vi "cl_serv_serv.vi"() -> ()   [LabVIEW 2015]
panel:
  out "String":string
  in  "close connection 4":bool
  in  "Control 4":bool
  in  "Slide 4":dbl(slide) scale=0.0..10.0
  out "number 4":dbl(slide) scale=0.0..10.0
  out "name:port 4":string
  out "ip:port23":string
  in  "close server 4":bool
  in  "Server Closed 4":string="The server VI closed the connection."
  in  "close connection 3":bool
  in  "Control 3":bool
  in  "Slide 3":dbl(slide) scale=0.0..10.0
  out "number 3":dbl(slide) scale=0.0..10.0
  out "name:port 3":string
  out "ip:port2 2":string
  in  "close server 3":bool
  in  "Server Closed 3":string="The server VI closed the connection."
  in  "close connection 2":bool
  in  "Control 2":bool
  in  "Slide 2":dbl(slide) scale=0.0..10.0
  out "number 2":dbl(slide) scale=0.0..10.0
  out "name:port 2":string
  out "ip:port2":string
  in  "close server 2":bool
  in  "Server Closed 2":string="The server VI closed the connection."
  in  "close server 1":bool
  out "ip:port 1":string
  out "name:port 1":string
  out "number 1":dbl(slide) scale=0.0..10.0
  in  "Slide 1":dbl(slide) scale=0.0..10.0
  in  "Control 1":bool
  in  "Server Closed 1":string="The server VI closed the connection."
  in  "close connection":bool
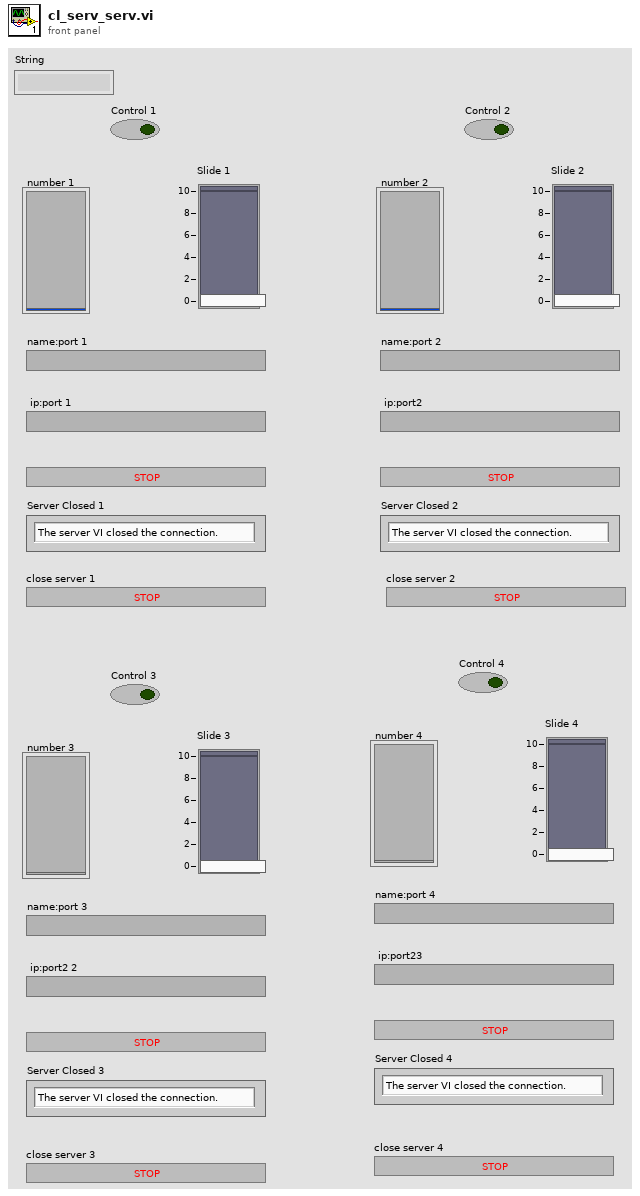
[diagram p1: front panel]
types:
  T1 = enum8{"Enabled", "Disabled", "Disabled and Grayed Out"}
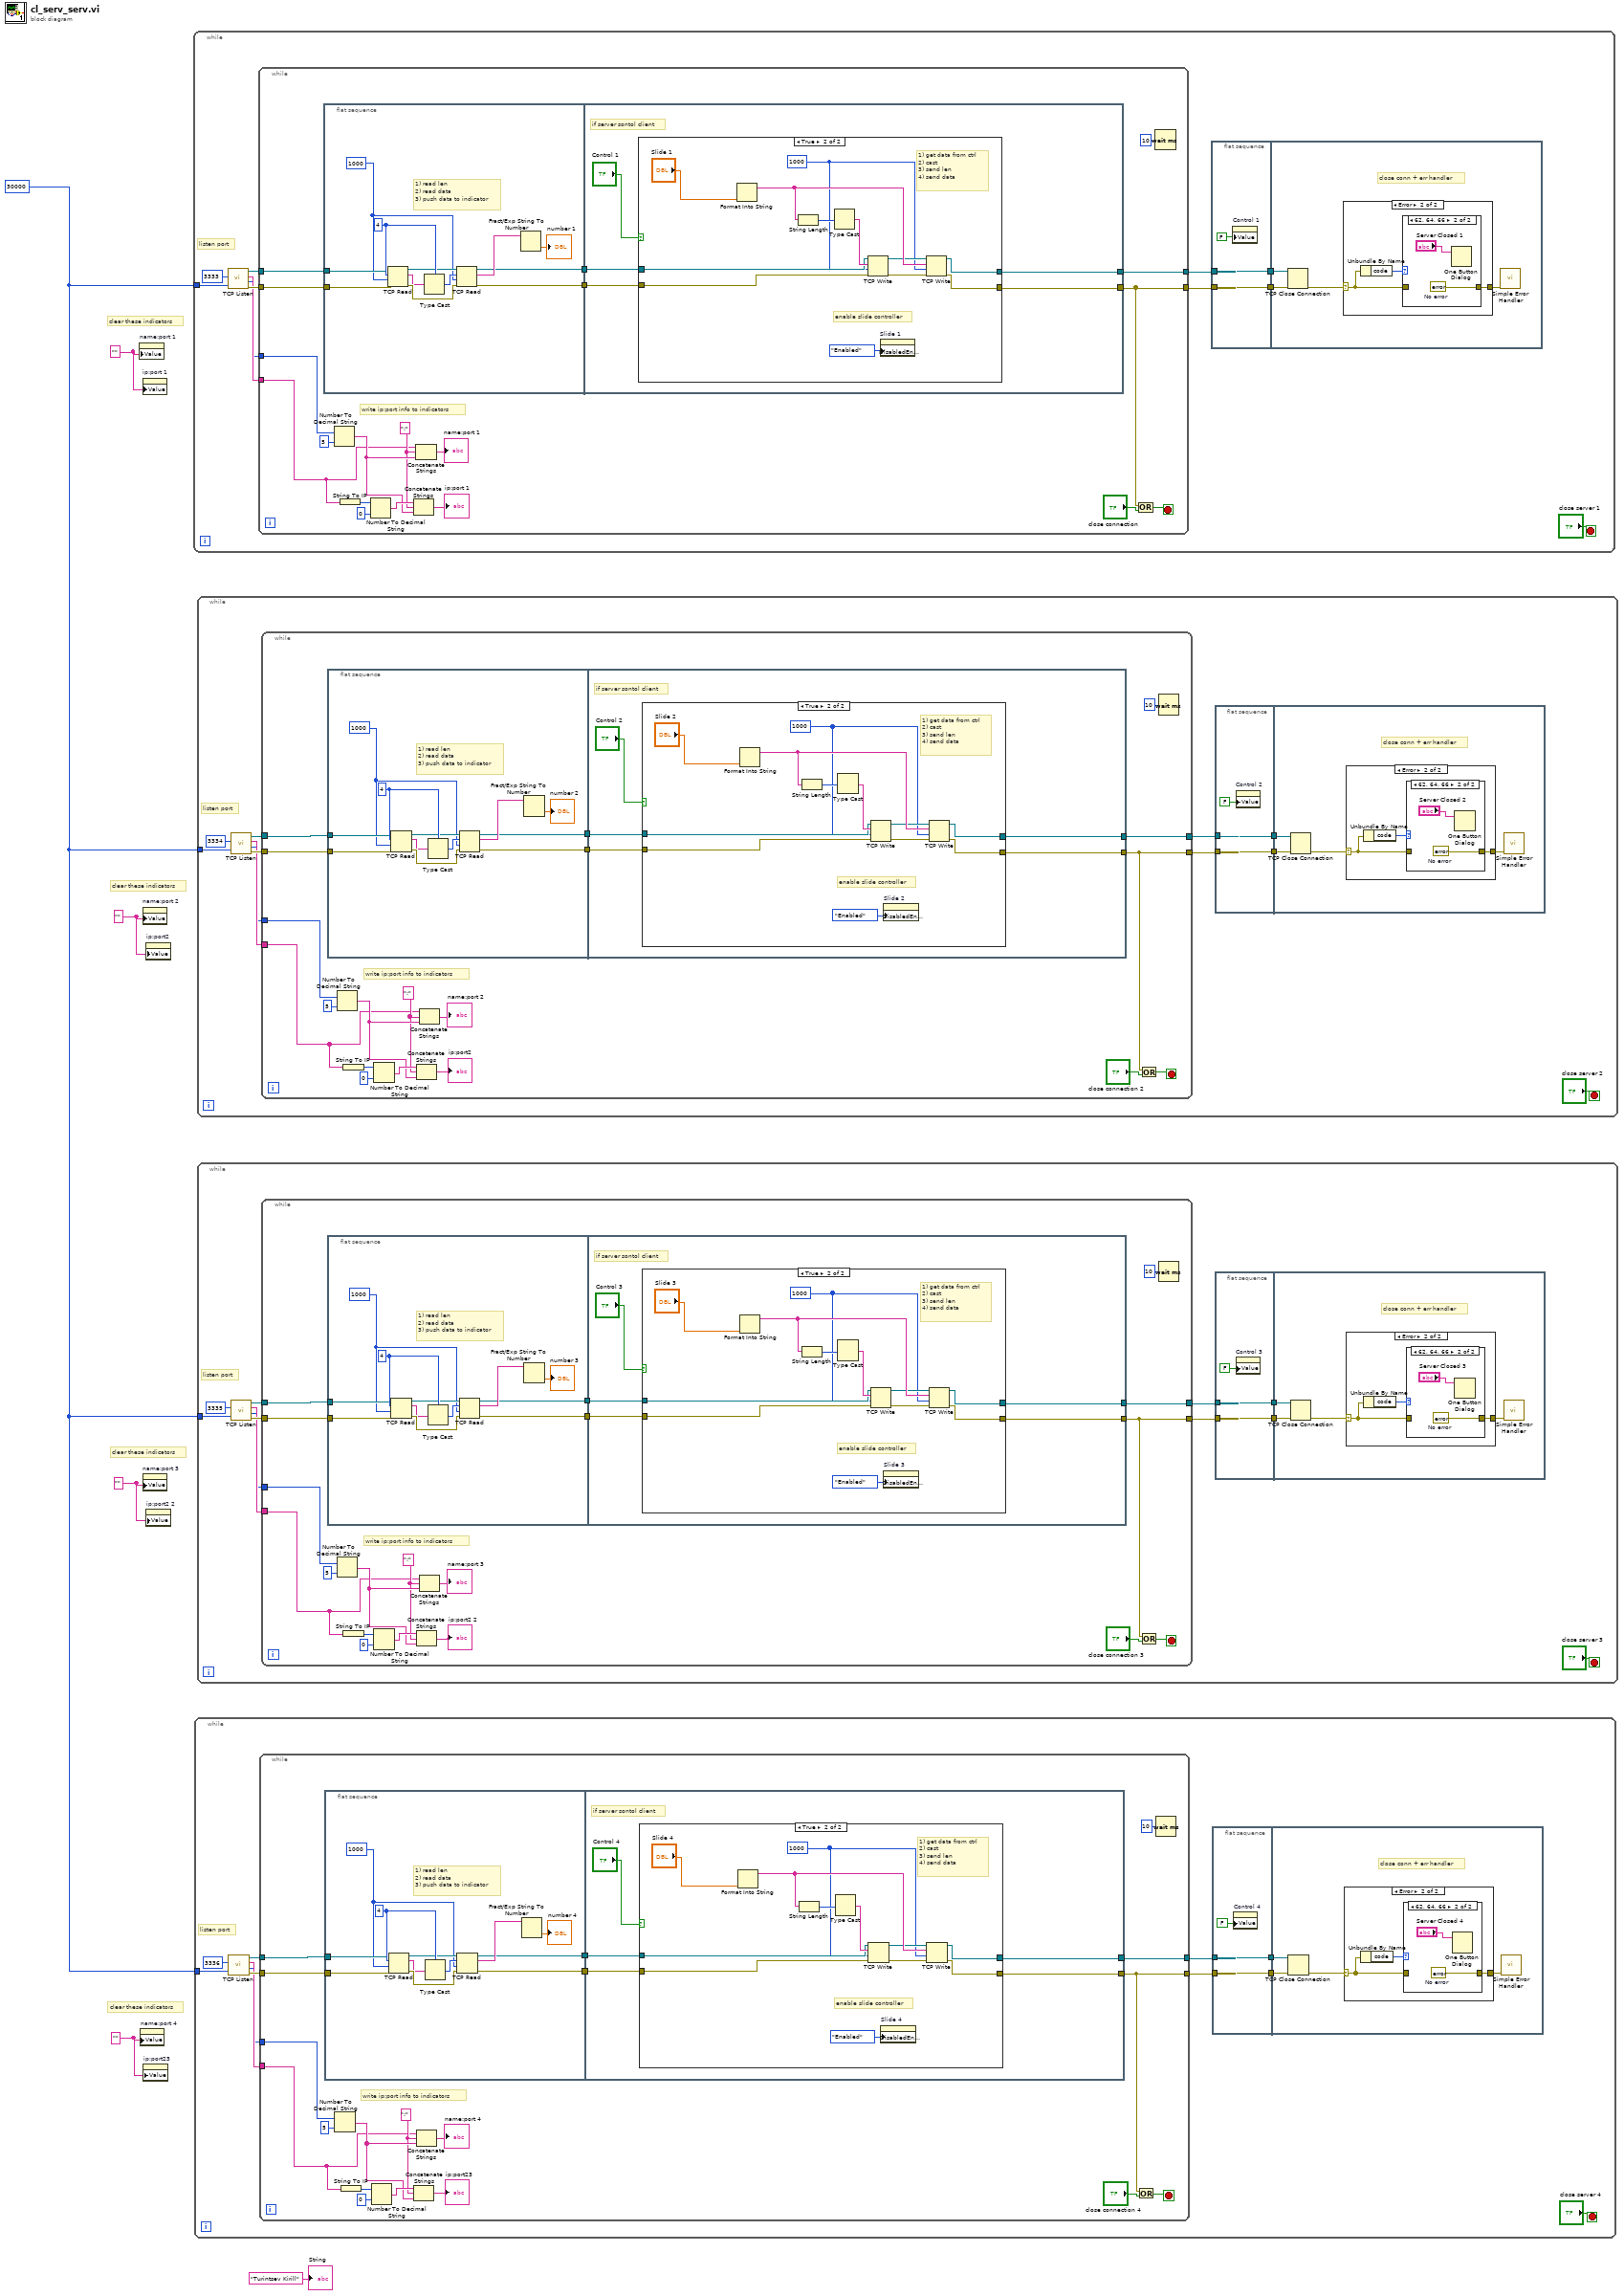
[diagram p0: block diagram]
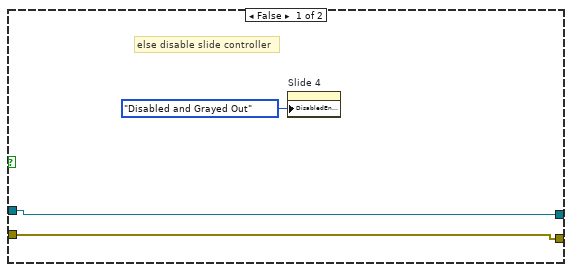
[diagram p4: hidden frame]
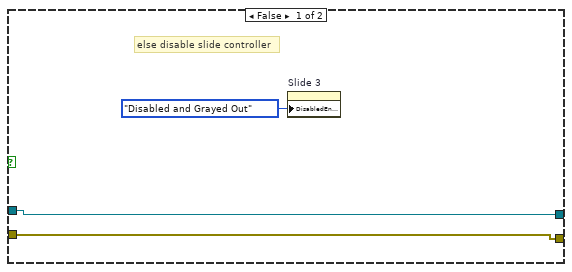
[diagram p7: hidden frame]
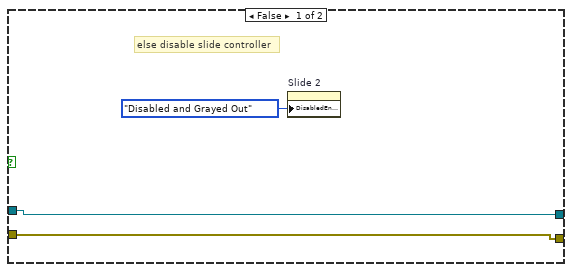
[diagram p10: hidden frame]
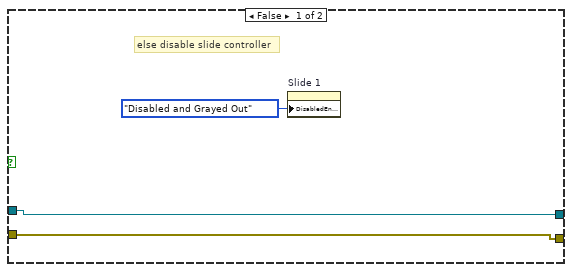
[diagram p13: hidden frame]
diagram:
  w3 = "" ("name:port 1")
  w4 = "" ("name:port 1")
  w5 = "" ("name:port 1")
  w2 = 30000 ("timeout ms (wait forever: -1)")
  w6 = "" ("name:port 1")
  # "clear these indicators"
  # "clear these indicators"
  # "clear these indicators"
  # "clear these indicators"
  n1 = property on="name:port 1" class="Str"("Value"=w6) -> ()  [unwired: 2 in, 2 out]
  n2 = property on="name:port 4" class="Str"("Value"=w3) -> ()  [unwired: 2 in, 2 out]
  n3 = property on="ip:port 1" class="Str"("Value"=w6) -> ()  [unwired: 2 in, 2 out]
  n4 = property on="name:port 2" class="Str"("Value"=w5) -> ()  [unwired: 2 in, 2 out]
  n5 = property on="name:port 3" class="Str"("Value"=w4) -> ()  [unwired: 2 in, 2 out]
  n6 = property on="ip:port23" class="Str"("Value"=w3) -> ()  [unwired: 2 in, 2 out]
  n7 = property on="ip:port2" class="Str"("Value"=w5) -> ()  [unwired: 2 in, 2 out]
  n8 = property on="ip:port2 2" class="Str"("Value"=w4) -> ()  [unwired: 2 in, 2 out]
  n9 = while {
    tunnel: w2 -> [w10]
    stop <- "close server 1" stop-if-true
    # "listen port"
    n10 = call <vilib>:"TCP Listen.vi"("timeout ms (wait forever: -1)"=w10, "port"=u16 3333) -> ("error out"=w14:errorcluster, "remote port"=w11:u16, "remote address"=w12:string, "connection ID"=w16:refnum<k5>)  [unwired: 5 in, 1 out]
    n11 = while {
      tunnel: w16 -> [w50]
      tunnel: [w46] -> w15
      tunnel: w14 -> [w49]
      tunnel: [w32] -> w13
      tunnel: w12 -> [w37]
      tunnel: w11 -> [w36]
      stop <- w34 stop-if-true
      w38 = ":" ("string")
      # "write ip:port info to indicators"
      n12 = flat-sequence {
        tunnel: w50 -> [w55]
        tunnel: w49 -> [w54]
        tunnel: [w53] -> w48
        tunnel: [w52] -> w47
        tunnel: w48 -> [w66]
        tunnel: w47 -> [w65]
        tunnel: [w64] -> w46
        tunnel: [w63] -> w32
        frame #0 {
          w51 = 1000 ("timeout ms (25000)")
          w59 = 4 ("bytes to read")
          # "1) read len\n2) read data\n3) push data to indicator"
          n13 = TCP Read(connection ID=w55, bytes to read=w59, error in (no error)=w54, 9:w51) -> (connection ID out=w56:refnum<k5>, data out=w57:string, error out=w60:errorcluster)  [unwired: 1 in]
          n14 = Type Cast(type=w59, x=w57) -> (*(type *) &x=w58:i32)
          n15 = TCP Read(connection ID=w56, bytes to read=w58, error in (no error)=w60, 9:w51) -> (connection ID out=w53:refnum<k5>, data out=w61:string, error out=w52:errorcluster)  [unwired: 1 in]
          n16 = Fract/Exp String To Number(string=w61) -> (number=→"number 1":dbl)  [unwired: 3 in, 1 out]
        }
        frame #1 {
          # "if server sontol client"
          n17 = case shown="True" "Control 1" {
            tunnel: w66 -> [w70 w76]
            tunnel: w65 -> [w69 w75]
            tunnel: [w70 w74] -> w64
            tunnel: [w69 w73] -> w63
            frame False {
              # "else disable slide controller"
              n18 = property on="Slide 1" class="Slide (strict)"("DisabledEnum"=T1."Disabled and Grayed Out" ("Disabled")) -> ()  [unwired: 2 in, 2 out]
            }
            frame True {
              w71 = 1000 ("timeout ms (25000)")
              # "1) get data from ctrl\n2) cast\n3) send len\n4) send data"
              # "enable slide controller"
              n19 = Format Into String("Slide 1") -> (resulting string=w82:string)  [unwired: 3 in, 1 out]
              n20 = String Length(string=w82) -> (length=w79:i32)
              n21 = Type Cast(x=w79) -> (*(type *) &x=w80:string)  [unwired: 1 out]
              n22 = TCP Write(connection ID=w76, data in=w80, error in (no error)=w75, 9:w71) -> (connection ID out=w77:refnum<k5>, error out=w78:errorcluster)  [unwired: 1 out]
              n23 = property on="Slide 1" class="Slide (strict)"("DisabledEnum"=T1."Enabled" ("Disabled")) -> ()  [unwired: 2 in, 2 out]
              n24 = TCP Write(connection ID=w77, data in=w82, error in (no error)=w78, 9:w71) -> (connection ID out=w74:refnum<k5>, error out=w73:errorcluster)  [unwired: 1 out]
            }
          }
        }
      }
      n25 = Number To Decimal String(number=w36, width (-)=i16 5) -> (decimal integer string=w40:string)
      n26 = String To IP(1:w37) -> (0:w43:u32)
      n27 = Number To Decimal String(number=w43, width (-)=i16 0) -> (decimal integer string=w41:string)
      n28 = Concatenate Strings(w41, w38, w40) -> (→"ip:port 1":string)
      n29 = Concatenate Strings(w37, w38, w40) -> (→"name:port 1":string)
      n30 = Or(x=w32, y="close connection") -> (x .or. y?=w34:bool)
      n31 = Wait (ms)(milliseconds to wait=u32 10) -> ()  [unwired: 1 out]
    }
    n32 = flat-sequence {
      tunnel: w13 -> [w19]
      tunnel: w15 -> [w20]
      tunnel: [w20] -> w8
      tunnel: [w19] -> w7
      tunnel: w8 -> [w24]
      tunnel: w7 -> [w22]
      frame #0 {
        n33 = property on="Control 1" class="Bool (strict)"("Value"=FALSE ("Control 1")) -> ()  [unwired: 2 in, 2 out]
      }
      frame #1 {
        # "close conn + err handler"
        n34 = TCP Close Connection(connection ID=w24, error in (no error)=w22) -> (error out=w21:errorcluster)  [unwired: 1 in, 1 out]
        n35 = case shown="Error" w21 {
          selector: w21 -> [w25 w27]
          tunnel: [w25 w26] -> w23
          frame No Error {
          }
          frame Error {
            n36 = Unbundle By Name(w27) -> ("code"=w28:i32)
            n37 = case shown="62, 64, 66" w28 {
              tunnel: w27 -> [w29 _]
              tunnel: [w29 w31] -> w26
              frame Default {
              }
              frame 62, 64, 66 {
                w31 = errorcluster {"status"=FALSE, "code"=0, "source"=""}  # No error
                n38 = One Button Dialog(message="Server Closed 1") -> ()  [unwired: 1 in, 1 out]
              }
            }
          }
        }
        n39 = call <vilib>:"Simple Error Handler.vi"("error in (no error)"=w23) -> ()  [unwired: 1 in, 8 out]
      }
    }
  }
  n40 = while {
    tunnel: w2 -> [w86]
    stop <- "close server 4" stop-if-true
    # "listen port"
    n41 = call <vilib>:"TCP Listen.vi"("timeout ms (wait forever: -1)"=w86, "port"=u16 3336) -> ("error out"=w90:errorcluster, "remote port"=w87:u16, "remote address"=w88:string, "connection ID"=w92:refnum<k5>)  [unwired: 5 in, 1 out]
    n42 = while {
      tunnel: w92 -> [w126]
      tunnel: [w122] -> w91
      tunnel: w90 -> [w125]
      tunnel: [w108] -> w89
      tunnel: w88 -> [w113]
      tunnel: w87 -> [w112]
      stop <- w110 stop-if-true
      w114 = ":" ("string")
      # "write ip:port info to indicators"
      n43 = flat-sequence {
        tunnel: w126 -> [w131]
        tunnel: w125 -> [w130]
        tunnel: [w129] -> w124
        tunnel: [w128] -> w123
        tunnel: w124 -> [w142]
        tunnel: w123 -> [w141]
        tunnel: [w140] -> w122
        tunnel: [w139] -> w108
        frame #0 {
          w127 = 1000 ("timeout ms (25000)")
          w135 = 4 ("bytes to read")
          # "1) read len\n2) read data\n3) push data to indicator"
          n44 = TCP Read(connection ID=w131, bytes to read=w135, error in (no error)=w130, 9:w127) -> (connection ID out=w132:refnum<k5>, data out=w133:string, error out=w136:errorcluster)  [unwired: 1 in]
          n45 = Type Cast(type=w135, x=w133) -> (*(type *) &x=w134:i32)
          n46 = TCP Read(connection ID=w132, bytes to read=w134, error in (no error)=w136, 9:w127) -> (connection ID out=w129:refnum<k5>, data out=w137:string, error out=w128:errorcluster)  [unwired: 1 in]
          n47 = Fract/Exp String To Number(string=w137) -> (number=→"number 4":dbl)  [unwired: 3 in, 1 out]
        }
        frame #1 {
          # "if server sontol client"
          n48 = case shown="True" "Control 4" {
            tunnel: w142 -> [w146 w152]
            tunnel: w141 -> [w145 w151]
            tunnel: [w146 w150] -> w140
            tunnel: [w145 w149] -> w139
            frame False {
              # "else disable slide controller"
              n49 = property on="Slide 4" class="Slide (strict)"("DisabledEnum"=T1."Disabled and Grayed Out" ("Disabled")) -> ()  [unwired: 2 in, 2 out]
            }
            frame True {
              w147 = 1000 ("timeout ms (25000)")
              # "1) get data from ctrl\n2) cast\n3) send len\n4) send data"
              # "enable slide controller"
              n50 = Format Into String("Slide 4") -> (resulting string=w158:string)  [unwired: 3 in, 1 out]
              n51 = String Length(string=w158) -> (length=w155:i32)
              n52 = Type Cast(x=w155) -> (*(type *) &x=w156:string)  [unwired: 1 out]
              n53 = TCP Write(connection ID=w152, data in=w156, error in (no error)=w151, 9:w147) -> (connection ID out=w153:refnum<k5>, error out=w154:errorcluster)  [unwired: 1 out]
              n54 = property on="Slide 4" class="Slide (strict)"("DisabledEnum"=T1."Enabled" ("Disabled")) -> ()  [unwired: 2 in, 2 out]
              n55 = TCP Write(connection ID=w153, data in=w158, error in (no error)=w154, 9:w147) -> (connection ID out=w150:refnum<k5>, error out=w149:errorcluster)  [unwired: 1 out]
            }
          }
        }
      }
      n56 = Number To Decimal String(number=w112, width (-)=i16 5) -> (decimal integer string=w116:string)
      n57 = String To IP(1:w113) -> (0:w119:u32)
      n58 = Number To Decimal String(number=w119, width (-)=i16 0) -> (decimal integer string=w117:string)
      n59 = Concatenate Strings(w117, w114, w116) -> (→"ip:port23":string)
      n60 = Concatenate Strings(w113, w114, w116) -> (→"name:port 4":string)
      n61 = Or(x=w108, y="close connection 4") -> (x .or. y?=w110:bool)
      n62 = Wait (ms)(milliseconds to wait=u32 10) -> ()  [unwired: 1 out]
    }
    n63 = flat-sequence {
      tunnel: w89 -> [w95]
      tunnel: w91 -> [w96]
      tunnel: [w96] -> w84
      tunnel: [w95] -> w83
      tunnel: w84 -> [w100]
      tunnel: w83 -> [w98]
      frame #0 {
        n64 = property on="Control 4" class="Bool (strict)"("Value"=FALSE ("Control 1")) -> ()  [unwired: 2 in, 2 out]
      }
      frame #1 {
        # "close conn + err handler"
        n65 = TCP Close Connection(connection ID=w100, error in (no error)=w98) -> (error out=w97:errorcluster)  [unwired: 1 in, 1 out]
        n66 = case shown="Error" w97 {
          selector: w97 -> [w101 w103]
          tunnel: [w101 w102] -> w99
          frame No Error {
          }
          frame Error {
            n67 = Unbundle By Name(w103) -> ("code"=w104:i32)
            n68 = case shown="62, 64, 66" w104 {
              tunnel: w103 -> [w105 _]
              tunnel: [w105 w107] -> w102
              frame Default {
              }
              frame 62, 64, 66 {
                w107 = errorcluster {"status"=FALSE, "code"=0, "source"=""}  # No error
                n69 = One Button Dialog(message="Server Closed 4") -> ()  [unwired: 1 in, 1 out]
              }
            }
          }
        }
        n70 = call <vilib>:"Simple Error Handler.vi"("error in (no error)"=w99) -> ()  [unwired: 1 in, 8 out]
      }
    }
  }
  n71 = while {
    tunnel: w2 -> [w162]
    stop <- "close server 2" stop-if-true
    # "listen port"
    n72 = call <vilib>:"TCP Listen.vi"("timeout ms (wait forever: -1)"=w162, "port"=u16 3334) -> ("error out"=w166:errorcluster, "remote port"=w163:u16, "remote address"=w164:string, "connection ID"=w168:refnum<k5>)  [unwired: 5 in, 1 out]
    n73 = while {
      tunnel: w168 -> [w202]
      tunnel: [w198] -> w167
      tunnel: w166 -> [w201]
      tunnel: [w184] -> w165
      tunnel: w164 -> [w189]
      tunnel: w163 -> [w188]
      stop <- w186 stop-if-true
      w190 = ":" ("string")
      # "write ip:port info to indicators"
      n74 = flat-sequence {
        tunnel: w202 -> [w207]
        tunnel: w201 -> [w206]
        tunnel: [w205] -> w200
        tunnel: [w204] -> w199
        tunnel: w200 -> [w218]
        tunnel: w199 -> [w217]
        tunnel: [w216] -> w198
        tunnel: [w215] -> w184
        frame #0 {
          w203 = 1000 ("timeout ms (25000)")
          w211 = 4 ("bytes to read")
          # "1) read len\n2) read data\n3) push data to indicator"
          n75 = TCP Read(connection ID=w207, bytes to read=w211, error in (no error)=w206, 9:w203) -> (connection ID out=w208:refnum<k5>, data out=w209:string, error out=w212:errorcluster)  [unwired: 1 in]
          n76 = Type Cast(type=w211, x=w209) -> (*(type *) &x=w210:i32)
          n77 = TCP Read(connection ID=w208, bytes to read=w210, error in (no error)=w212, 9:w203) -> (connection ID out=w205:refnum<k5>, data out=w213:string, error out=w204:errorcluster)  [unwired: 1 in]
          n78 = Fract/Exp String To Number(string=w213) -> (number=→"number 2":dbl)  [unwired: 3 in, 1 out]
        }
        frame #1 {
          # "if server sontol client"
          n79 = case shown="True" "Control 2" {
            tunnel: w218 -> [w222 w228]
            tunnel: w217 -> [w221 w227]
            tunnel: [w222 w226] -> w216
            tunnel: [w221 w225] -> w215
            frame False {
              # "else disable slide controller"
              n80 = property on="Slide 2" class="Slide (strict)"("DisabledEnum"=T1."Disabled and Grayed Out" ("Disabled")) -> ()  [unwired: 2 in, 2 out]
            }
            frame True {
              w223 = 1000 ("timeout ms (25000)")
              # "1) get data from ctrl\n2) cast\n3) send len\n4) send data"
              # "enable slide controller"
              n81 = Format Into String("Slide 2") -> (resulting string=w234:string)  [unwired: 3 in, 1 out]
              n82 = String Length(string=w234) -> (length=w231:i32)
              n83 = Type Cast(x=w231) -> (*(type *) &x=w232:string)  [unwired: 1 out]
              n84 = TCP Write(connection ID=w228, data in=w232, error in (no error)=w227, 9:w223) -> (connection ID out=w229:refnum<k5>, error out=w230:errorcluster)  [unwired: 1 out]
              n85 = property on="Slide 2" class="Slide (strict)"("DisabledEnum"=T1."Enabled" ("Disabled")) -> ()  [unwired: 2 in, 2 out]
              n86 = TCP Write(connection ID=w229, data in=w234, error in (no error)=w230, 9:w223) -> (connection ID out=w226:refnum<k5>, error out=w225:errorcluster)  [unwired: 1 out]
            }
          }
        }
      }
      n87 = Number To Decimal String(number=w188, width (-)=i16 5) -> (decimal integer string=w192:string)
      n88 = String To IP(1:w189) -> (0:w195:u32)
      n89 = Number To Decimal String(number=w195, width (-)=i16 0) -> (decimal integer string=w193:string)
      n90 = Concatenate Strings(w193, w190, w192) -> (→"ip:port2":string)
      n91 = Concatenate Strings(w189, w190, w192) -> (→"name:port 2":string)
      n92 = Or(x=w184, y="close connection 2") -> (x .or. y?=w186:bool)
      n93 = Wait (ms)(milliseconds to wait=u32 10) -> ()  [unwired: 1 out]
    }
    n94 = flat-sequence {
      tunnel: w165 -> [w171]
      tunnel: w167 -> [w172]
      tunnel: [w172] -> w160
      tunnel: [w171] -> w159
      tunnel: w160 -> [w176]
      tunnel: w159 -> [w174]
      frame #0 {
        n95 = property on="Control 2" class="Bool (strict)"("Value"=FALSE ("Control 1")) -> ()  [unwired: 2 in, 2 out]
      }
      frame #1 {
        # "close conn + err handler"
        n96 = TCP Close Connection(connection ID=w176, error in (no error)=w174) -> (error out=w173:errorcluster)  [unwired: 1 in, 1 out]
        n97 = case shown="Error" w173 {
          selector: w173 -> [w177 w179]
          tunnel: [w177 w178] -> w175
          frame No Error {
          }
          frame Error {
            n98 = Unbundle By Name(w179) -> ("code"=w180:i32)
            n99 = case shown="62, 64, 66" w180 {
              tunnel: w179 -> [w181 _]
              tunnel: [w181 w183] -> w178
              frame Default {
              }
              frame 62, 64, 66 {
                w183 = errorcluster {"status"=FALSE, "code"=0, "source"=""}  # No error
                n100 = One Button Dialog(message="Server Closed 2") -> ()  [unwired: 1 in, 1 out]
              }
            }
          }
        }
        n101 = call <vilib>:"Simple Error Handler.vi"("error in (no error)"=w175) -> ()  [unwired: 1 in, 8 out]
      }
    }
  }
  n102 = while {
    tunnel: w2 -> [w238]
    stop <- "close server 3" stop-if-true
    # "listen port"
    n103 = call <vilib>:"TCP Listen.vi"("timeout ms (wait forever: -1)"=w238, "port"=u16 3335) -> ("error out"=w242:errorcluster, "remote port"=w239:u16, "remote address"=w240:string, "connection ID"=w244:refnum<k5>)  [unwired: 5 in, 1 out]
    n104 = while {
      tunnel: w244 -> [w278]
      tunnel: [w274] -> w243
      tunnel: w242 -> [w277]
      tunnel: [w260] -> w241
      tunnel: w240 -> [w265]
      tunnel: w239 -> [w264]
      stop <- w262 stop-if-true
      w266 = ":" ("string")
      # "write ip:port info to indicators"
      n105 = flat-sequence {
        tunnel: w278 -> [w283]
        tunnel: w277 -> [w282]
        tunnel: [w281] -> w276
        tunnel: [w280] -> w275
        tunnel: w276 -> [w294]
        tunnel: w275 -> [w293]
        tunnel: [w292] -> w274
        tunnel: [w291] -> w260
        frame #0 {
          w279 = 1000 ("timeout ms (25000)")
          w287 = 4 ("bytes to read")
          # "1) read len\n2) read data\n3) push data to indicator"
          n106 = TCP Read(connection ID=w283, bytes to read=w287, error in (no error)=w282, 9:w279) -> (connection ID out=w284:refnum<k5>, data out=w285:string, error out=w288:errorcluster)  [unwired: 1 in]
          n107 = Type Cast(type=w287, x=w285) -> (*(type *) &x=w286:i32)
          n108 = TCP Read(connection ID=w284, bytes to read=w286, error in (no error)=w288, 9:w279) -> (connection ID out=w281:refnum<k5>, data out=w289:string, error out=w280:errorcluster)  [unwired: 1 in]
          n109 = Fract/Exp String To Number(string=w289) -> (number=→"number 3":dbl)  [unwired: 3 in, 1 out]
        }
        frame #1 {
          # "if server sontol client"
          n110 = case shown="True" "Control 3" {
            tunnel: w294 -> [w298 w304]
            tunnel: w293 -> [w297 w303]
            tunnel: [w298 w302] -> w292
            tunnel: [w297 w301] -> w291
            frame False {
              # "else disable slide controller"
              n111 = property on="Slide 3" class="Slide (strict)"("DisabledEnum"=T1."Disabled and Grayed Out" ("Disabled")) -> ()  [unwired: 2 in, 2 out]
            }
            frame True {
              w299 = 1000 ("timeout ms (25000)")
              # "1) get data from ctrl\n2) cast\n3) send len\n4) send data"
              # "enable slide controller"
              n112 = Format Into String("Slide 3") -> (resulting string=w310:string)  [unwired: 3 in, 1 out]
              n113 = String Length(string=w310) -> (length=w307:i32)
              n114 = Type Cast(x=w307) -> (*(type *) &x=w308:string)  [unwired: 1 out]
              n115 = TCP Write(connection ID=w304, data in=w308, error in (no error)=w303, 9:w299) -> (connection ID out=w305:refnum<k5>, error out=w306:errorcluster)  [unwired: 1 out]
              n116 = property on="Slide 3" class="Slide (strict)"("DisabledEnum"=T1."Enabled" ("Disabled")) -> ()  [unwired: 2 in, 2 out]
              n117 = TCP Write(connection ID=w305, data in=w310, error in (no error)=w306, 9:w299) -> (connection ID out=w302:refnum<k5>, error out=w301:errorcluster)  [unwired: 1 out]
            }
          }
        }
      }
      n118 = Number To Decimal String(number=w264, width (-)=i16 5) -> (decimal integer string=w268:string)
      n119 = String To IP(1:w265) -> (0:w271:u32)
      n120 = Number To Decimal String(number=w271, width (-)=i16 0) -> (decimal integer string=w269:string)
      n121 = Concatenate Strings(w269, w266, w268) -> (→"ip:port2 2":string)
      n122 = Concatenate Strings(w265, w266, w268) -> (→"name:port 3":string)
      n123 = Or(x=w260, y="close connection 3") -> (x .or. y?=w262:bool)
      n124 = Wait (ms)(milliseconds to wait=u32 10) -> ()  [unwired: 1 out]
    }
    n125 = flat-sequence {
      tunnel: w241 -> [w247]
      tunnel: w243 -> [w248]
      tunnel: [w248] -> w236
      tunnel: [w247] -> w235
      tunnel: w236 -> [w252]
      tunnel: w235 -> [w250]
      frame #0 {
        n126 = property on="Control 3" class="Bool (strict)"("Value"=FALSE ("Control 1")) -> ()  [unwired: 2 in, 2 out]
      }
      frame #1 {
        # "close conn + err handler"
        n127 = TCP Close Connection(connection ID=w252, error in (no error)=w250) -> (error out=w249:errorcluster)  [unwired: 1 in, 1 out]
        n128 = case shown="Error" w249 {
          selector: w249 -> [w253 w255]
          tunnel: [w253 w254] -> w251
          frame No Error {
          }
          frame Error {
            n129 = Unbundle By Name(w255) -> ("code"=w256:i32)
            n130 = case shown="62, 64, 66" w256 {
              tunnel: w255 -> [w257 _]
              tunnel: [w257 w259] -> w254
              frame Default {
              }
              frame 62, 64, 66 {
                w259 = errorcluster {"status"=FALSE, "code"=0, "source"=""}  # No error
                n131 = One Button Dialog(message="Server Closed 3") -> ()  [unwired: 1 in, 1 out]
              }
            }
          }
        }
        n132 = call <vilib>:"Simple Error Handler.vi"("error in (no error)"=w251) -> ()  [unwired: 1 in, 8 out]
      }
    }
  }
  "String" <- "Turintsev Kirill" ("String")
